vi "ApplyScalePost.vi"(8 "error in (no error)":errorcluster, 10 "Y Array":sgl[](array[numeric]), 11 "Thermocouple in":refnum<class "Thermocouple.lvclass">) -> (0 "error out":errorcluster, 2 "Y Array":sgl[](array[numeric]), 3 "Thermocouple out":refnum<class "Thermocouple.lvclass">)   [LabVIEW 2012, in "Measurement Channels.lvlib" / "Thermocouple.lvclass"]
uses:
  Thermocouple.lvclass
  Class Channel/Read Scale.vi
  Class Channel/Read Offset.vi
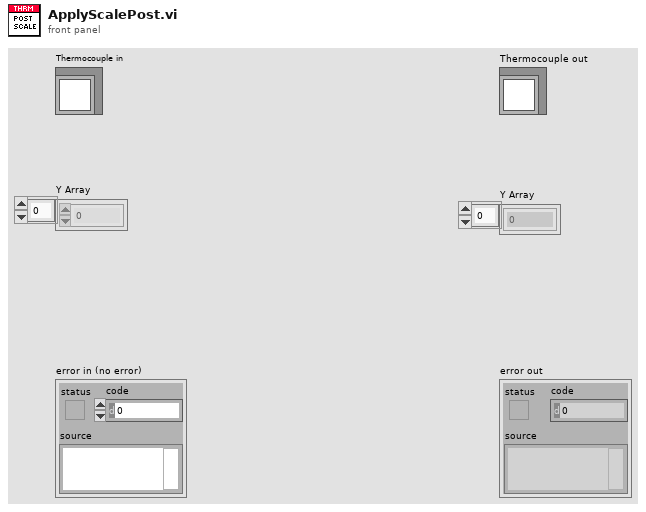
[diagram p1: front panel]
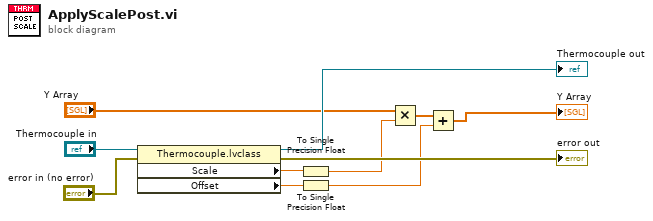
[diagram p0: block diagram]
diagram:
  n1 = property class="Thermocouple.lvclass"(reference="Thermocouple in", error in="error in (no error)") -> (reference out=→"Thermocouple out":refnum<class "Thermocouple.lvclass">, error out=→"error out":errorcluster, "Scale"=w4:dbl, "Offset"=w3:dbl)
  n2 = To Single Precision Float(number=w4) -> (single precision float=w2:sgl)
  n3 = To Single Precision Float(number=w3) -> (single precision float=w1:sgl)
  n4 = Multiply(x="Y Array", y=w2) -> (x*y=w7:sgl[])
  n5 = Add(x=w7, y=w1) -> (x+y=→"Y Array":sgl[])
